vi "Init time array.vi"(7 "DAQ":T1={"Data"={"Live"={"t0"=timestamp(0 s since 1904-01-01), "dt"=1.0, "Y"=[]}, "Accumulated"={"t0"=timestamp(0 s since 1904-01-01), "dt"=1.0, "Y"=[]}, "Averaged"={"t0"=timestamp(0 s since 1904-01-01), "dt"=1.0, "Y"=[]}, "data array"=[], "live time array"=[], "Live (decimated)"={"t0"=timestamp(0 s since 1904-01-01), "dt"=1.0, "Y"=[]}}, "Config"={"Input Config"=0, "Card"=enum."USB-6211", "100% Reflectance Standard (V)"=0.0, "Input Channel"="", "Average number of points"=0.0, "Trigger Level (V)"=0.0, "Rate (Hz)"=0, "End Time (s)"=0.0}, "Indicators"={"Final number of points"=0.0, "Number of samples"=0.0, "dt"=0.0, "Shots"=10, "Shot counter"=10, "Test counter"=10, "Background level (V)"=0.0, "DAQ task"="", "timestamp of data"=timestamp(0 s since 1904-01-01), "Test Type"=enum."A-Test"}} {"Config"."Input Config" items=["default"=-1, "RSE"=10083, "NRSE"=10078, "Differential"=10106, "Pseudodifferential"=12529]}, 8 "error in (no error)":errorcluster) -> (0 "error out":errorcluster, 5 "DAQ out":T1={"Data"={"Live"={"t0"=timestamp(0 s since 1904-01-01), "dt"=1.0, "Y"=[]}, "Accumulated"={"t0"=timestamp(0 s since 1904-01-01), "dt"=1.0, "Y"=[]}, "Averaged"={"t0"=timestamp(0 s since 1904-01-01), "dt"=1.0, "Y"=[]}, "data array"=[], "live time array"=[], "Live (decimated)"={"t0"=timestamp(0 s since 1904-01-01), "dt"=1.0, "Y"=[]}}, "Config"={"Input Config"=0, "Card"=enum."USB-6211", "100% Reflectance Standard (V)"=0.0, "Input Channel"="", "Average number of points"=0.0, "Trigger Level (V)"=0.0, "Rate (Hz)"=0, "End Time (s)"=0.0}, "Indicators"={"Final number of points"=0.0, "Number of samples"=0.0, "dt"=0.0, "Shots"=10, "Shot counter"=10, "Test counter"=10, "Background level (V)"=0.0, "DAQ task"="", "timestamp of data"=timestamp(0 s since 1904-01-01), "Test Type"=enum."A-Test"}} {"Config"."Input Config" items=["default"=-1, "RSE"=10083, "NRSE"=10078, "Differential"=10106, "Pseudodifferential"=12529]})   [LabVIEW 2017, in "DAQ.lvlib"]
uses:
  DAQ.lvlib
  Controls/Params.ctl
  Controls/DAQ Config.ctl
  Controls/DAQ Indicators.ctl
  System Control/CTLs/Test Type.ctl
  System Control/Main controller.lvlib
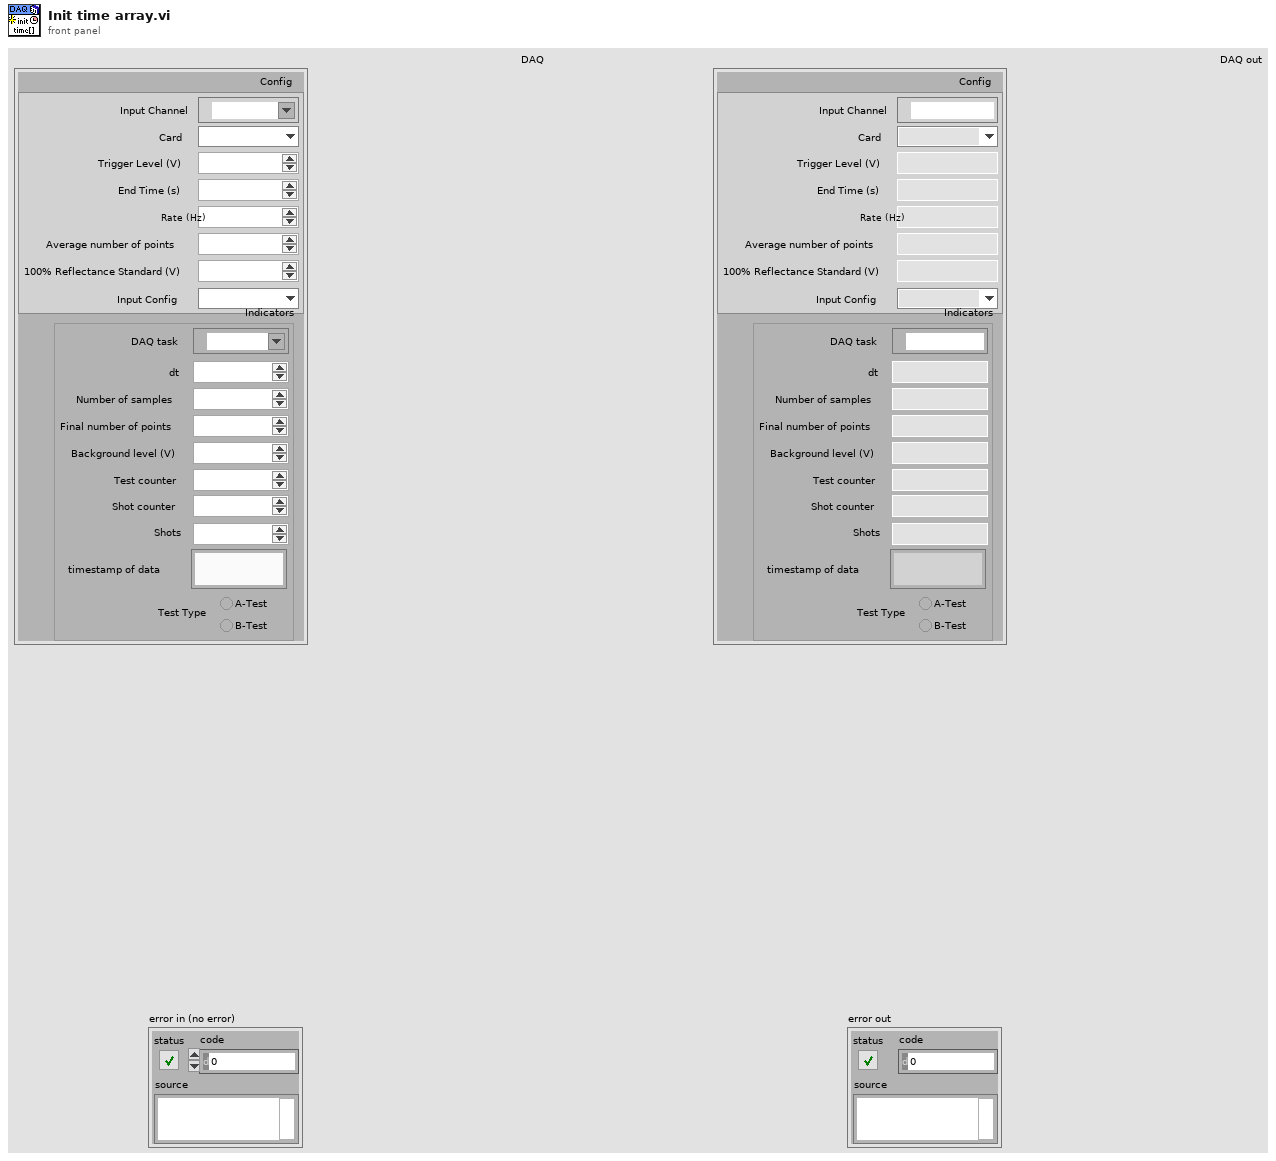
[diagram p1: front panel]
types:
  T1 = typedef "DAQ.lvlib/Params.ctl" = cluster{"Data":cluster{"Live":waveform(dbl), "Accumulated":waveform(dbl), "Averaged":waveform(dbl), "data array":dbl[], "live time array":dbl[], "Live (decimated)":waveform(dbl)}, "Config":T2, "Indicators":T3}
  T2 = typedef "DAQ.lvlib/DAQ Config.ctl" = cluster{"Input Config":i32, "Card":enum16{"USB-6211", "USB-6251", "USB-6361"}, "100% Reflectance Standard (V)":dbl, "Input Channel":tag, "Average number of points":dbl, "Trigger Level (V)":dbl, "Rate (Hz)":i32, "End Time (s)":dbl}
  T3 = typedef "DAQ.lvlib/DAQ Indicators.ctl" = cluster{"Final number of points":dbl, "Number of samples":dbl, "dt":dbl, "Shots":i32, "Shot counter":i32, "Test counter":i32, "Background level (V)":dbl, "DAQ task":refnum<k21>, "timestamp of data":timestamp, "Test Type":T4}
  T4 = typedef "Main controller.lvlib/Test Type.ctl" = enum32{"A-Test", "B-Test"}
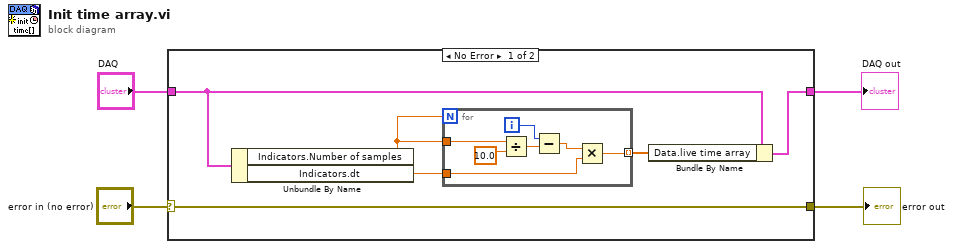
[diagram p0: block diagram]
diagram:
  n1 = case shown="No Error" "error in (no error)" {
    selector: "error in (no error)" -> [w5 w19]
    tunnel: "DAQ" -> [w10 w18]
    tunnel: [w9 w18] -> w3
    tunnel: [w5 w19] -> w1
    frame No Error {
      n2 = Unbundle By Name(w10) -> ("Indicators.Number of samples"=w8:dbl, "Indicators.dt"=w7:dbl)
      n3 = for {
        N: w8 -> [_]
        tunnel: [w13] -> w6 mode=indexing
        tunnel: w8 -> [w12]
        tunnel: w7 -> [w11]
        i -> [w17]
        n4 = Divide(x=w12, y=10.0) -> (x/y=w15:dbl)
        n5 = Subtract(x=w17, y=w15) -> (x-y=w14:dbl)
        n6 = Multiply(x=w14, y=w11) -> (x*y=w13:dbl)
      }
      n7 = Bundle By Name(cluster=w10, "Data.live time array"=w6) -> (w9:T1)
    }
    frame Error {
    }
  }
  "error out" <- w1
  "DAQ out" <- w3
